vi "20TDewarMonitor.vi"() -> ()   [LabVIEW 2016]
uses:
  Utility/Monitor Communication/Gustav/20T_Dewar_Cluster.ctl
  Instrument_Setup.vi
  Global/Global Variables/Data_Display_global.vi
  Equipment/Mercury iXX/Public/Libraries/Heater/Open/Open Heater Device.vi
  Equipment/Mercury iXX/Public/Libraries/Heater/Signals/Read/Power (Read).vi
  Equipment/Mercury iXX/Public/Libraries/Pressure/Open/Open Pressure Device.vi
  Equipment/Mercury iXX/Public/Libraries/Pressure/Signals/Read/Pressure (Read).vi
  Equipment/Mercury iXX/Public/Libraries/Temperature/Signals/Read/Status Heater (Read).vi
  Utility/Monitor Communication/sub-vis/20TDewar_Open_Queue.vi
  Utility/Monitor Communication/sub-vis/20TDewar_Check_Queue.vi
  Equipment/Mercury iXX/Mercury iXX.lvlib
  Equipment/Mercury iXX/Public/Libraries/Pressure.lvlib
  Equipment/Mercury iXX/Public/Libraries/Heater.lvlib
panel:
  out "20T-Dewar-Cluster":T1={"Dewar Heater (%)"=0.0, "D-Heater (%) Display"=3.4572, "D-Heater SP"=0.0, "Set D-Heater SP"=FALSE, "Change D-Heater Status"=FALSE, "Dewar Pressure"=0.0, "Dewar heater manual"=FALSE} {"Dewar Pressure" format="%4_5f"; "D-Heater (%) Display" format="%4_5f"; "Dewar Heater (%)" scale=0.0..100.0}
  in  "local error":errorcluster
  # "Dewar Heater (%)"
  # "Dewar Pressure"
  # "Setpoint"
  # "20T Dewar"
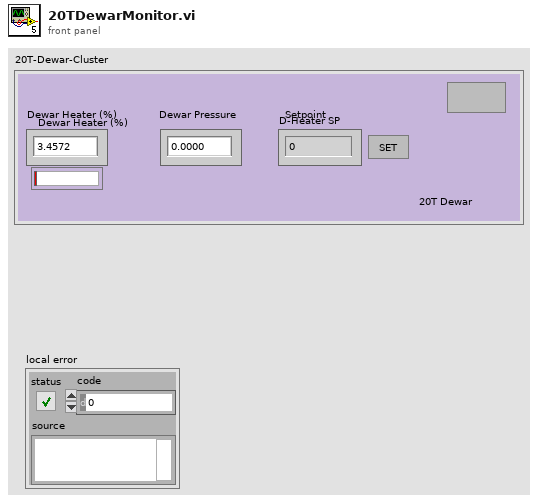
[diagram p1: front panel]
types:
  T1 = typedef "20T_Dewar_Cluster.ctl" = cluster{"Dewar Heater (%)":dbl, "D-Heater (%) Display":dbl, "D-Heater SP":dbl, "Set D-Heater SP":bool, "Change D-Heater Status":bool, "Dewar Pressure":dbl, "Dewar heater manual":bool}
  T2 = typedef "Mercury iXX.lvlib/Mercury Reference.ctl" = cluster{"Comms":refnum<visa-resource-name>, "Device ID":string[], "Comms Layer":T3, "Command":string, "Query reference":T4}
  T3 = typedef "Mercury iXX.lvlib/Comms Transport Layer.ctl" = enum16{"Ethernet TCP/IP", "USB", "ISOBus - RS-232", "GPIB"}
  T4 = typedef "Mercury iXX.lvlib/Query Dynamic Reference.ctl" = refnum<vi>
  T5 = typedef "Mercury iXX.lvlib/Unit String.ctl" = string
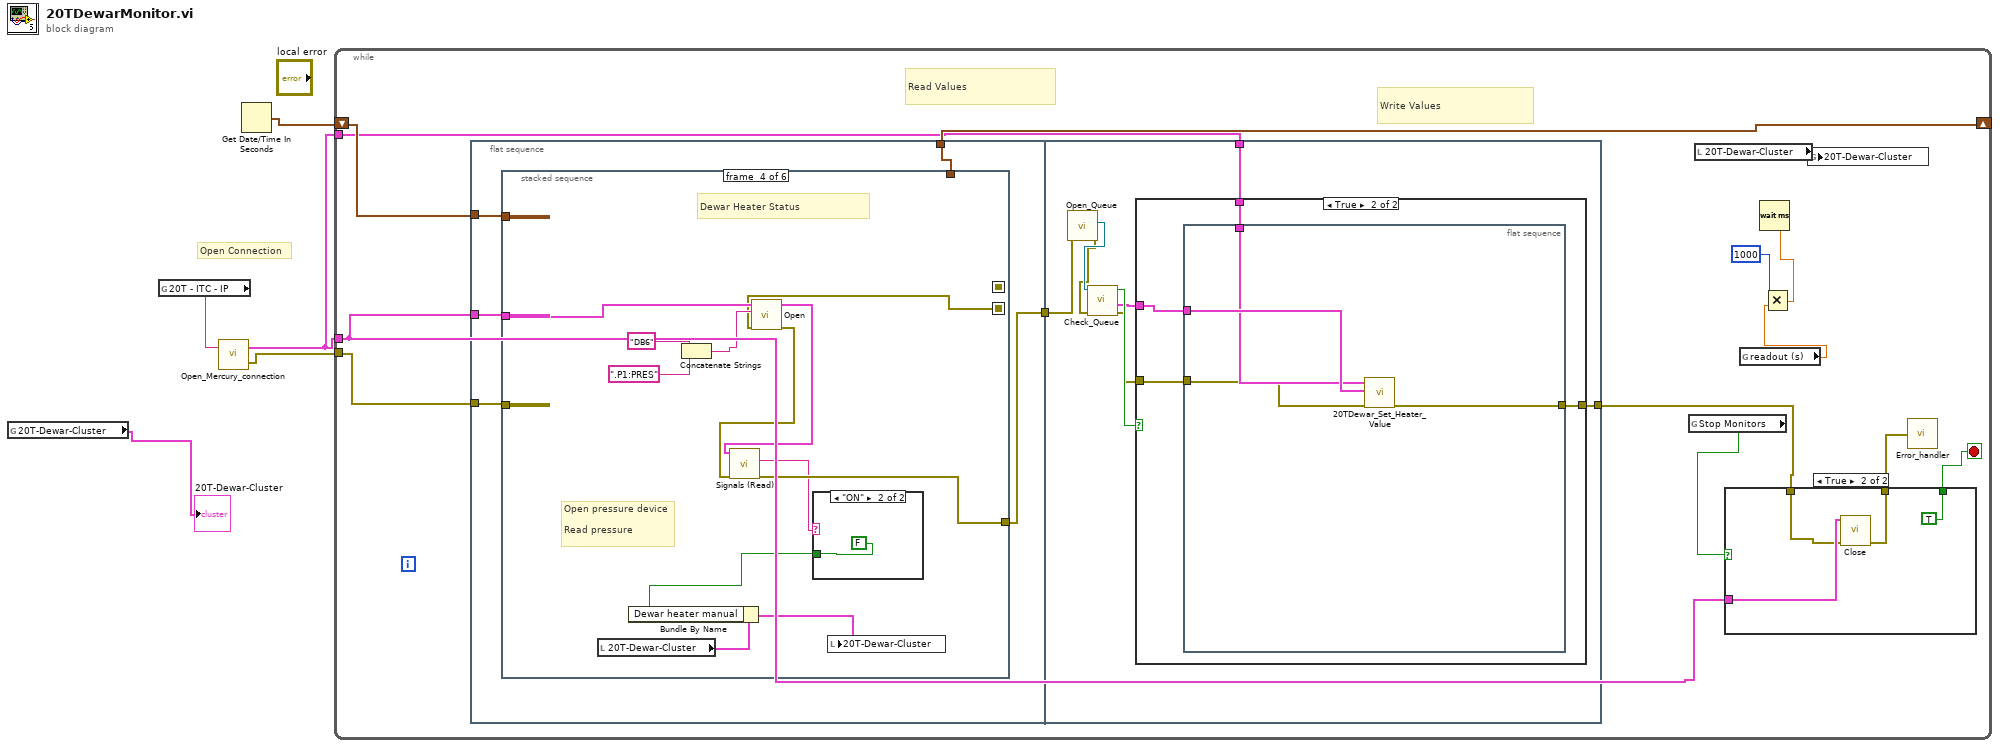
[diagram p0: block diagram]
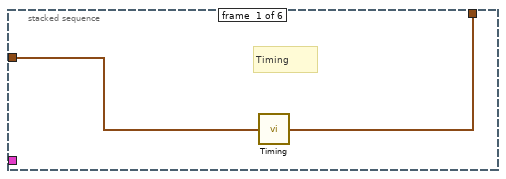
[diagram p2: hidden frame]
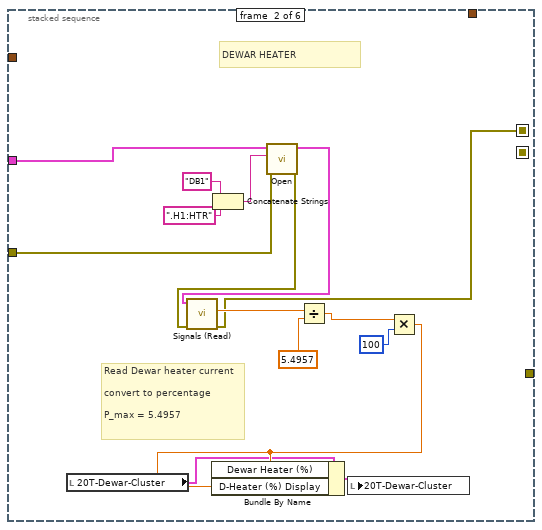
[diagram p3: hidden frame]
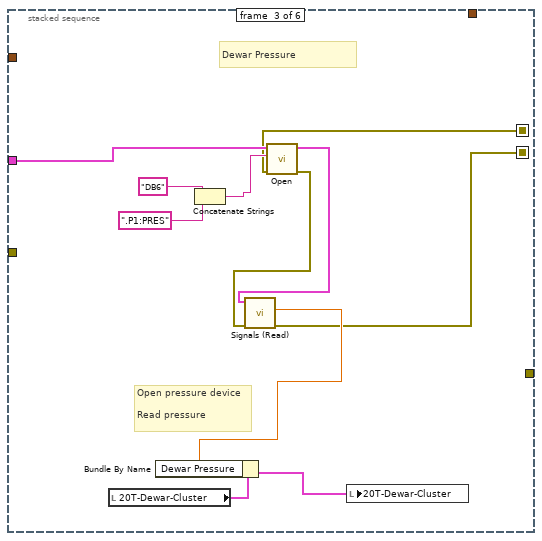
[diagram p4: hidden frame]
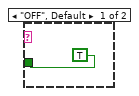
[diagram p5: hidden frame]
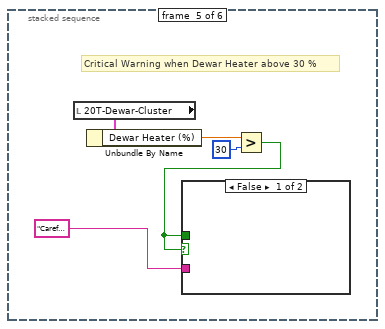
[diagram p6: hidden frame]
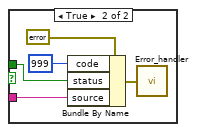
[diagram p7: hidden frame]
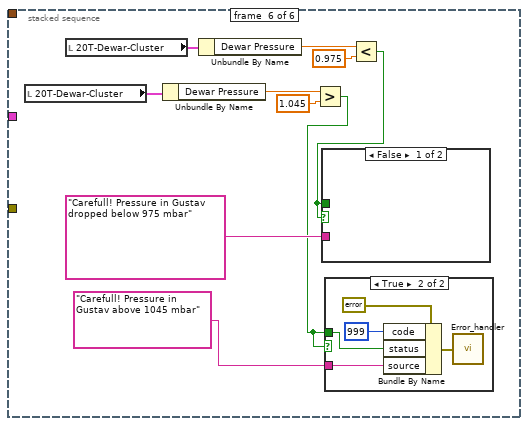
[diagram p8: hidden frame]
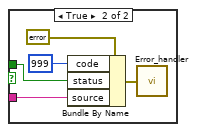
[diagram p10: hidden frame]
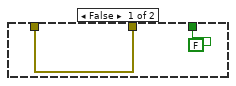
[diagram p12: hidden frame]
diagram:
  # "Open Connection"
  n1 = global read "Data_Display_global.vi" "20T-Dewar-Cluster"() -> (→"20T-Dewar-Cluster":T1)
  n2 = global read "Instrument_Setup.vi" "20T - ITC - IP"() -> (w5:string)
  n3 = call "Open_Mercury_connection.vi"("IP Address"=w5) -> ("error out"=w2:errorcluster, "Mercury Reference Out"=w1:T2)  [unwired: 1 in]
  n4 = Get Date/Time In Seconds() -> (seconds since 1Jan1904=w4:timestamp)
  n5 = while {
    tunnel: w1 -> [w10]
    tunnel: w2 -> [w19]
    shift-right: [w11] -> _
    shift-left: w4 -> [w12]
    tunnel: w1 -> [w7]
    stop <- w15 stop-if-true
    # "Write Values"
    # "Read Values"
    n6 = flat-sequence {
      tunnel: w19 -> [w24]
      tunnel: w10 -> [w23]
      tunnel: w12 -> [w22]
      tunnel: [w21] -> w11
      tunnel: [w20] -> w8
      tunnel: w8 -> [w103]
      tunnel: w7 -> [w99]
      tunnel: [w97] -> w6
      frame #0 {
        n7 = stacked-sequence {
          seq-local: [_ w30 _ _ _ _] -> [_ _ w42 _ _ _]
          seq-local: [_ _ w45 _ _ _] -> [_ _ _ w53 _ _]
          tunnel: w23 -> [_ w39 w52 w64 _ _]
          tunnel: w24 -> [_ w37 _ _ _ _]
          tunnel: [_ _ _ w58 _ _] -> w20
          tunnel: w22 -> [w26 _ _ _ _ _]
          tunnel: [w25 _ _ _ _ _] -> w21
          frame #0 {
            # "Timing"
            n8 = call "Timing.vi"("start time (s)"=w26) -> ("last reading (s)"=w25:timestamp)
          }
          frame #1 {
            # "DEWAR HEATER"
            # "Read Dewar heater current\n\nconvert to percentage\n\nP_max = 5.4957"
            n9 = local read "20T-Dewar-Cluster"() -> (w28:T1)
            n10 = Concatenate Strings("DB1", ".H1:HTR" ("Device Identifier")) -> (w38:string)
            n11 = call-poly "Open.vi"("error in (no error)"=w37, "Device Identifier"=w38, "Mercury Reference In"=w39) -> ("error out"=w31:errorcluster, "Mercury Reference Out"=w32:T2)  [unwired: 1 in, 6 out]
            n12 = call-poly "Signals (Read).vi"("error in"=w31, "Mercury Reference In"=w32) -> ("error out"=w30:errorcluster, "Power"=w33:dbl)  [unwired: 5 in, 3 out]
            n13 = Divide(x=w33, y=5.4957) -> (x/y=w35:dbl)
            n14 = Multiply(x=w35, y=100) -> (x*y=w29:dbl)
            n15 = Bundle By Name(cluster=w28, "Dewar Heater (%)"=w29, "D-Heater (%) Display"=w29) -> (w27:T1)
            n16 = local write "20T-Dewar-Cluster"(w27) -> ()
          }
          frame #2 {
            # "Open pressure device\n\nRead pressure"
            # "Dewar Pressure"
            n17 = local read "20T-Dewar-Cluster"() -> (w44:T1)
            n18 = Concatenate Strings("DB6", ".P1:PRES" ("Device Identifier")) -> (w47:string)
            n19 = call-poly "Open.vi"("error in (no error)"=w42, "Device Identifier"=w47, "Mercury Reference In"=w52) -> ("error out"=w50:errorcluster, "Mercury Reference Out"=w51:T2)  [unwired: 1 in, 6 out]
            n20 = call-poly "Signals (Read).vi"("error in"=w50, "Mercury Reference In"=w51) -> ("error out"=w45:errorcluster, "Temperature"=w46:dbl)  [unwired: 5 in, 3 out]
            n21 = Bundle By Name(cluster=w44, "Dewar Pressure"=w46) -> (w43:T1)
            n22 = local write "20T-Dewar-Cluster"(w43) -> ()
          }
          frame #3 {
            # "Open pressure device\n\nRead pressure"
            # "Dewar Heater Status"
            n23 = local read "20T-Dewar-Cluster"() -> (w55:T1)
            n24 = Concatenate Strings("DB6", ".P1:PRES" ("Device Identifier")) -> (w59:string)
            n25 = call-poly "Open.vi"("error in (no error)"=w53, "Device Identifier"=w59, "Mercury Reference In"=w64) -> ("error out"=w62:errorcluster, "Mercury Reference Out"=w63:T2)  [unwired: 1 in, 6 out]
            n26 = call-poly "Signals (Read).vi"("error in"=w62, "Mercury Reference In"=w63) -> ("error out"=w58:errorcluster, "State"=w57:T5)  [unwired: 6 in, 2 out]
            n27 = case shown="\"ON\"" w57 {
              tunnel: [TRUE FALSE] -> w56
              frame "OFF", Default {
              }
              frame "ON" {
              }
            }
            n28 = Bundle By Name(cluster=w55, "Dewar heater manual"=w56) -> (w54:T1)
            n29 = local write "20T-Dewar-Cluster"(w54) -> ()
          }
          frame #4 {
            # "Critical Warning when Dewar Heater above 30 %"
            n30 = local read "20T-Dewar-Cluster"() -> (w68:T1)
            n31 = Unbundle By Name(w68) -> ("Dewar Heater (%)"=w67:dbl)
            n32 = Greater?(x=w67, y=30) -> (0:w69:bool)
            n33 = case shown="False" w69 {
              tunnel: w69 -> [_ w75]
              tunnel: "Carefull! Bath heater above 30 %. Check for leak or empty dewar" -> [_ w74]
              frame False {
              }
              frame True {
                n34 = Bundle By Name(cluster=errorcluster {"status"=FALSE, "code"=0, "source"=""} ("error constant"), "code"=999, "status"=w75, "source"=w74) -> (w73:errorcluster)
                n35 = call "Error_handler.vi"("error constant"=w73) -> ()
              }
            }
          }
          frame #5 {
            n36 = local read "20T-Dewar-Cluster"() -> (w79:T1)
            n37 = local read "20T-Dewar-Cluster"() -> (w86:T1)
            n38 = Unbundle By Name(w79) -> ("Dewar Pressure"=w81:dbl)
            n39 = Unbundle By Name(w86) -> ("Dewar Pressure"=w85:dbl)
            n40 = Greater?(x=w81, y=1.045) -> (0:w78:bool)
            n41 = case shown="True" w78 {
              tunnel: w78 -> [_ w90]
              tunnel: "Carefull! Pressure in Gustav above 1045 mbar" -> [_ w89]
              frame False {
              }
              frame True {
                n42 = Bundle By Name(cluster=errorcluster {"status"=FALSE, "code"=0, "source"=""} ("error constant"), "code"=999, "status"=w90, "source"=w89) -> (w88:errorcluster)
                n43 = call "Error_handler.vi"("error constant"=w88) -> ()
              }
            }
            n44 = Less?(x=w85, y=0.975) -> (x < y?=w83:bool)
            n45 = case shown="False" w83 {
              tunnel: w83 -> [_ w95]
              tunnel: "Carefull! Pressure in Gustav dropped below 975 mbar" -> [_ w94]
              frame False {
              }
              frame True {
                n46 = Bundle By Name(cluster=errorcluster {"status"=FALSE, "code"=0, "source"=""} ("error constant"), "code"=999, "status"=w95, "source"=w94) -> (w93:errorcluster)
                n47 = call "Error_handler.vi"("error constant"=w93) -> ()
              }
            }
          }
        }
      }
      frame #1 {
        n48 = call-poly "Open_Queue.vi"("error in (no error)"=w103) -> ("error out"=w102:errorcluster, "queue out"=w104:refnum<queue>)  [unwired: 9 in]
        n49 = call-poly "Check_Queue.vi"("error in (no error)"=w102, "queue"=w104) -> ("error out"=w98:errorcluster, "Control"=w100:T1, "New Entries?"=w101:bool)  [unwired: 6 in]
        n50 = case shown="True" w101 {
          tunnel: w100 -> [_ w109]
          tunnel: w99 -> [_ w108]
          tunnel: w98 -> [w105 w107]
          tunnel: [w105 w106] -> w97
          frame False {
          }
          frame True {
            n51 = flat-sequence {
              tunnel: w109 -> [w113]
              tunnel: w108 -> [w112]
              tunnel: w107 -> [w111]
              tunnel: [w110] -> w106
              frame #0 {
                n52 = call "20TDewar_Set_Heater_Value.vi"("error in (no error)"=w111, "20T-Dewar-Cluster"=w113, "Mercury Reference In"=w112) -> ("error out"=w110:errorcluster)  [unwired: 8 in]
              }
            }
          }
        }
      }
    }
    n53 = global read "Data_Display_global.vi" "Stop Monitors"() -> (w13:bool)
    n54 = local read "20T-Dewar-Cluster"() -> (w9:T1)
    n55 = case shown="True" w13 {
      tunnel: w10 -> [_ w119]
      tunnel: [w114 w116] -> w14
      tunnel: [FALSE TRUE] -> w15
      tunnel: w6 -> [w114 w117]
      frame False {
      }
      frame True {
        n56 = call "Close.vi"("error in (no error)"=w117, "Mercury Reference"=w119) -> ("error out"=w116:errorcluster)  [unwired: 9 in]
      }
    }
    n57 = global read "Instrument_Setup.vi" "readout (s)"() -> (w18:dbl)
    n58 = Multiply(x=1000, y=w18) -> (x*y=w17:dbl)
    n59 = Wait (ms)(milliseconds to wait=w17) -> ()  [unwired: 1 out]
    n60 = global write "Data_Display_global.vi" "20T-Dewar-Cluster"(w9) -> ()
    n61 = call "Error_handler.vi"("error constant"=w14) -> ()
  }
